vi "4_1.vi"() -> ()   [LabVIEW 2020]
panel:
  out "Array 3":dbl[](array[numeric])=[100.0]
  out "Array 2":dbl[](array[numeric])=[100.0]
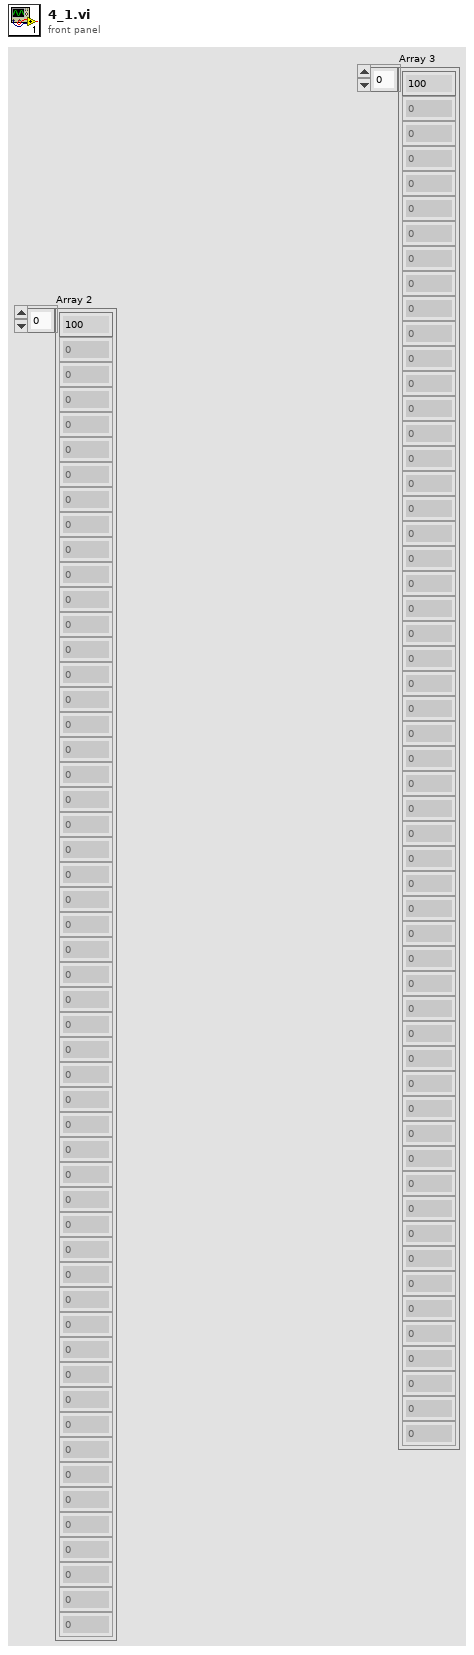
[diagram p1: front panel]
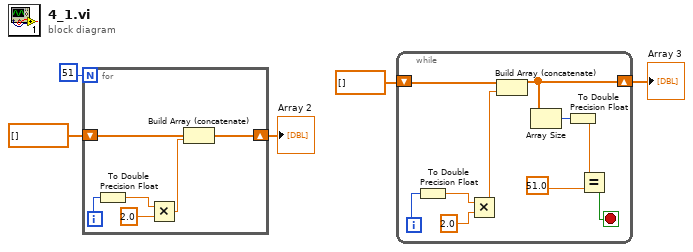
[diagram p0: block diagram]
diagram:
  n1 = for {
    N: 51 -> [_]
    shift-right: [w7] -> w3
    shift-left: dbl[] [] -> [w8]
    i -> [w10]
    n2 = To Double Precision Float(number=w10) -> (double precision float=w9:dbl)
    n3 = Multiply(x=w9, y=2.0) -> (x*y=w6:dbl)
    n4 = Build Array (concatenate)(w8, w6) -> (w7:dbl[])
  }
  "Array 2" <- w3
  n5 = while {
    shift-right: [w16] -> w1
    shift-left: dbl[] [] ("Array 3") -> [w18]
    i -> [w19]
    stop <- w13 stop-if-true
    n6 = To Double Precision Float(number=w19) -> (double precision float=w20:dbl)
    n7 = Multiply(x=w20, y=2.0) -> (x*y=w17:dbl)
    n8 = Build Array (concatenate)(w18, w17) -> (w16:dbl[])
    n9 = Array Size(array=w16) -> (size(s)=w14:i32)
    n10 = To Double Precision Float(number=w14) -> (double precision float=w12:dbl)
    n11 = Equal?(x=w12, y=51.0) -> (x = y?=w13:bool)
  }
  "Array 3" <- w1
